vi "SR830 query frequency.vi"(8 "error in (no error)":errorcluster, 11 "VISA resource name":refnum<visa-resource-name>) -> (0 "error out":errorcluster, 2 "frequency":dbl[unit], 3 "VISA resource name out":refnum<visa-resource-name>)   [LabVIEW 2017, in "SR830.lvlib"]
doc: "Reads the current frequency of the lock-in amplifier."
uses:
  SR830.lvlib
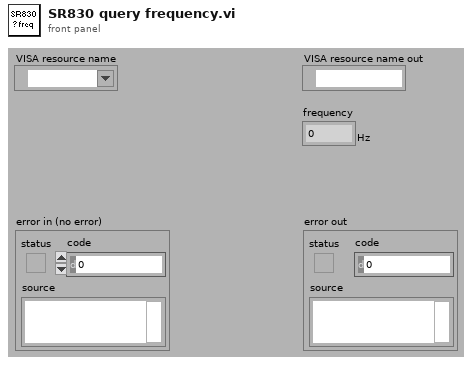
[diagram p1: front panel]
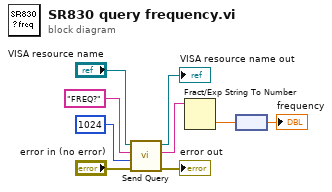
[diagram p0: block diagram]
diagram:
  n1 = call "Send Query.vi"("error in (no error)"="error in (no error)", "Bytes Count"=u32 1024 ("bytes to read (1000)"), "write buffer"="FREQ?", "VISA resource name"="VISA resource name") -> ("error out"=→"error out":errorcluster, "read buffer"=w1:string, "VISA resource name out"=→"VISA resource name out":refnum<visa-resource-name>)  [unwired: 5 in]
  n2 = Fract/Exp String To Number(string=w1) -> (number=w9:dbl)  [unwired: 4 out]
  n3 = node(w9) -> (→"frequency":dbl[unit])
